vi "sio flush.vi"(10 "func":i32, 11 "port":i32) -> (3 "function return":i32)   [LabVIEW 2012, in "PCOMM.lvlib"]
doc: "int WINAPI sio_flush(int port, int func);"
uses:
  PCOMM.lvlib
  #001 2018-09-10/Data/PCOMM.DLL
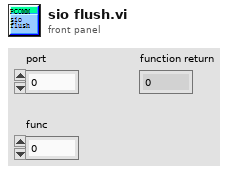
[diagram p1: front panel]
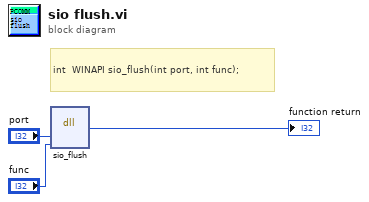
[diagram p0: block diagram]
diagram:
  # "int  WINAPI sio_flush(int port, int func);"
  n1 = dll-call lib="E:/ProJect/#008 ESDMonitor/#002 Labview/#001 2018-09-10/Data/PCOMM.*" fn="sio_flush"("port"="port", "func"="func") -> (→"function return":i32)  [unwired: 5 in, 2 out]
